vi "test Configuration Files Errors.vi"(8 "error in":errorcluster, 11 "TestCase in":refnum<class "Scripting.lvclass">) -> (0 "error out":errorcluster, 3 "TestCase out":refnum<class "Scripting.lvclass">)   [LabVIEW 2020, in "Scripting.lvclass"]
uses:
  Scripting.lvclass
  C:/dev/git/niveristand-custom-device-testing-tools/VeriStandScriptingTestCase/VeriStandScriptingTestCase.lvclass
  niveristand-custom-device-testing-tools/VeriStandScriptingTestCase/VeriStandScriptingTestCase.lvclass/VeriStandScriptingTestCase.ctl
  niveristand-custom-device-testing-tools/VeriStandScriptingTestCase/Read Target.vi
  Scripting/Constants.vi
  NationalInstruments.VeriStand.SystemDefinitionAPI
  <vilib>/addons/_JKI Toolkits/VI Tester/TestCase.llb/TestCase.lvclass
  Scripting/AIM MIL-STD-1553 Scripting.lvlib
  niveristand-custom-device-testing-tools/VeriStandTestUtilities/VeriStandTestUtilities.lvlib
  C:/Program Files (x86)/National Instruments/LabVIEW 2020/vi.lib/addons/_JKI Toolkits/VI Tester/TestCase.llb/TestCase.lvclass
  C:/dev/git/niveristand-aim-milStd1553-custom-device/Source/Custom Device Support/Tests/Unit/Scripting/Scripting.lvclass
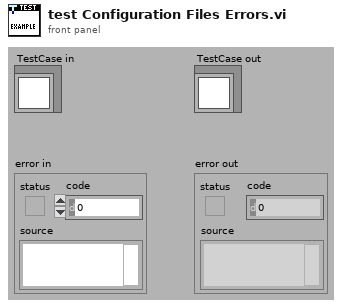
[diagram p1: front panel]
types:
  T1 = enum16{"open", "replace", "create", "open or create", "replace or create", "replace or create with confirmation"}
  T2 = typedef "Custom Device API.lvlib/Custom Device Item Ref.ctl" = u64
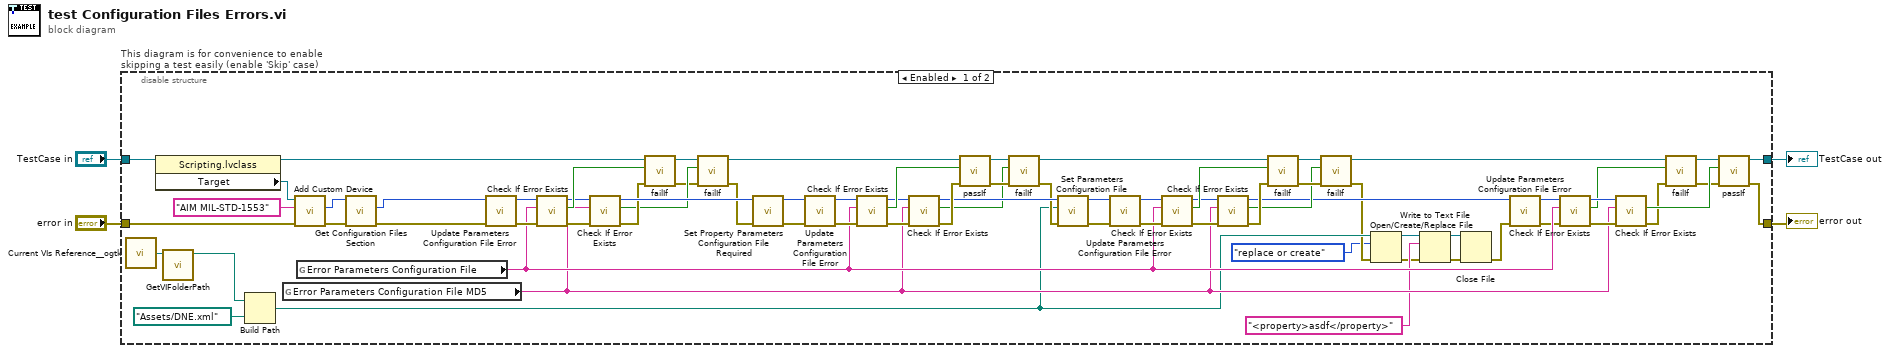
[diagram p0: block diagram]
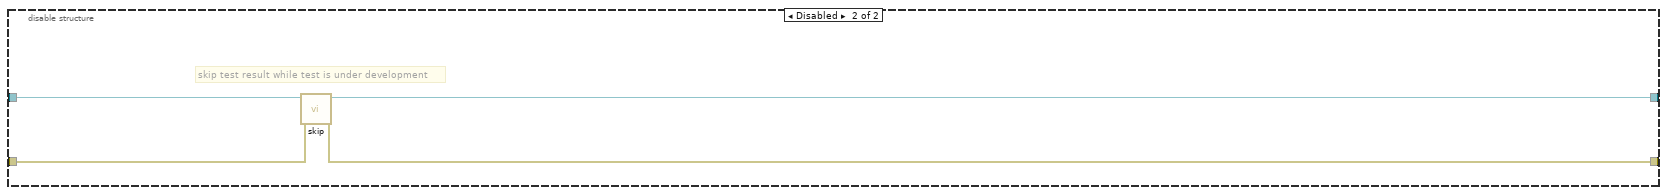
[diagram p2: hidden frame]
diagram:
  n1 = disable-structure "This diagram is for convenience to enable skipping a test easily (enable 'Skip' case)" shown="Enabled" {
    disable-tunnel: "TestCase in" -> [w75 w81]
    disable-tunnel: [w20 w79] -> w1
    disable-tunnel: [w19 w80] -> w3
    disable-tunnel: "error in" -> [w77 w78]
    frame Enabled {
      n2 = call <userlib>:"Current VIs Reference__ogtk.vi"() -> ("Current VI's reference"=w73:refnum<vi>)  [unwired: 5 in]
      n3 = property on="Property Node" class="Scripting.lvclass"(reference=w75) -> (reference out=w72:refnum<class "Scripting.lvclass">, "Target"=w74:refnum<k24>)  [unwired: 1 in, 1 out]
      n4 = call "GetVIFolderPath.vi"("VI Reference in"=w73) -> ("VI Folder Path out"=w59:path)  [unwired: 9 in, 1 out]
      n5 = Build Path(base path=w59, name or relative path=path "Assets/DNE.xml" ("hardware configuration file path")) -> (appended path=w11:path)
      n6 = global read "Constants.vi" "Error Parameters Configuration File MD5"() -> (w21:string)
      n7 = call "Add Custom Device.vi"("error in"=w77, "name"="AIM MIL-STD-1553", "target in"=w74) -> ("error out"=w67:errorcluster, "Ballard MIL-STD 1553 custom device"=w68:T2)  [unwired: 6 in, 1 out]
      n8 = global read "Constants.vi" "Error Parameters Configuration File"() -> (w22:string)
      n9 = call "Get Configuration Files Section.vi"("error in"=w67, "custom device in"=w68) -> ("error out"=w5:errorcluster, "configuration files section"=w6:T2)  [unwired: 6 in, 2 out]
      n10 = call "Update Parameters Configuration File Error.vi"("error in"=w5, "configuration files ref in"=w6) -> ("error out"=w71:errorcluster, "configuration files ref out"=w70:T2)  [unwired: 8 in]
      n11 = call "Check If Error Exists.vi"("error in"=w71, "error key"=w22, "section ref in"=w70) -> ("error out"=w53:errorcluster, "error exists?"=w69:bool, "section ref out"=w54:T2)  [unwired: 6 in]
      n12 = call "Check If Error Exists.vi"("error in"=w53, "error key"=w21, "section ref in"=w54) -> ("error out"=w51:errorcluster, "error exists?"=w50:bool, "section ref out"=w52:T2)  [unwired: 6 in]
      n13 = call-dynamic "failIf.vi"("error in (no error)"=w51, "fail"=w69, "TestCase in"=w72) -> ("error out"=w49:errorcluster, "TestCase out"=w48:refnum<class "Scripting.lvclass">)  [unwired: 7 in]
      n14 = call-dynamic "failIf.vi"("error in (no error)"=w49, "fail"=w50, "TestCase in"=w48) -> ("error out"=w47:errorcluster, "TestCase out"=w46:refnum<class "Scripting.lvclass">)  [unwired: 7 in]
      n15 = call "Set Property Parameters Configuration File Required.vi"("error in"=w47, "configuration files ref"=w52) -> ("error out"=w63:errorcluster, "configuration files ref out"=w64:T2)  [unwired: 8 in]
      n16 = call "Update Parameters Configuration File Error.vi"("error in"=w63, "configuration files ref in"=w64) -> ("error out"=w65:errorcluster, "configuration files ref out"=w66:T2)  [unwired: 8 in]
      n17 = call "Check If Error Exists.vi"("error in"=w65, "error key"=w22, "section ref in"=w66) -> ("error out"=w45:errorcluster, "error exists?"=w62:bool, "section ref out"=w44:T2)  [unwired: 6 in]
      n18 = call "Check If Error Exists.vi"("error in"=w45, "error key"=w21, "section ref in"=w44) -> ("error out"=w43:errorcluster, "error exists?"=w37:bool, "section ref out"=w42:T2)  [unwired: 6 in]
      n19 = call-dynamic "passIf.vi"("error in (no error)"=w43, "pass"=w62, "TestCase in"=w46) -> ("error out"=w40:errorcluster, "TestCase out"=w41:refnum<class "Scripting.lvclass">)  [unwired: 7 in]
      n20 = call-dynamic "failIf.vi"("error in (no error)"=w40, "fail"=w37, "TestCase in"=w41) -> ("error out"=w39:errorcluster, "TestCase out"=w38:refnum<class "Scripting.lvclass">)  [unwired: 7 in]
      n21 = call "Set Parameters Configuration File.vi"("error in"=w39, "parameters configuration file path"=w11, "Ballard MIL-STD 1553 custom device in"=w42) -> ("error out"=w56:errorcluster, "Ballard MIL-STD 1553 custom device out"=w57:T2)  [unwired: 7 in]
      n22 = call "Update Parameters Configuration File Error.vi"("error in"=w56, "configuration files ref in"=w57) -> ("error out"=w61:errorcluster, "configuration files ref out"=w60:T2)  [unwired: 8 in]
      n23 = call "Check If Error Exists.vi"("error in"=w61, "error key"=w22, "section ref in"=w60) -> ("error out"=w36:errorcluster, "error exists?"=w55:bool, "section ref out"=w35:T2)  [unwired: 6 in]
      n24 = call "Check If Error Exists.vi"("error in"=w36, "error key"=w21, "section ref in"=w35) -> ("error out"=w34:errorcluster, "error exists?"=w31:bool, "section ref out"=w15:T2)  [unwired: 6 in]
      n25 = call-dynamic "failIf.vi"("error in (no error)"=w34, "fail"=w55, "TestCase in"=w38) -> ("error out"=w32:errorcluster, "TestCase out"=w33:refnum<class "Scripting.lvclass">)  [unwired: 7 in]
      n26 = call-dynamic "failIf.vi"("error in (no error)"=w32, "fail"=w31, "TestCase in"=w33) -> ("error out"=w10:errorcluster, "TestCase out"=w23:refnum<class "Scripting.lvclass">)  [unwired: 7 in]
      n27 = Open/Create/Replace File(file path (use dialog)=w11, error in=w10, operation (0:open)=T1."replace or create") -> (refnum out=w9:refnum<file>, error out=w8:errorcluster)  [unwired: 3 in, 1 out]
      n28 = Write to Text File(file (use dialog)=w9, text="<property>asdf</property>", error in=w8) -> (refnum out=w17:refnum<file>, error out=w16:errorcluster)  [unwired: 1 in, 1 out]
      n29 = Close File(refnum=w17, error in=w16) -> (error out=w14:errorcluster)  [unwired: 1 out]
      n30 = call "Update Parameters Configuration File Error.vi"("error in"=w14, "configuration files ref in"=w15) -> ("error out"=w12:errorcluster, "configuration files ref out"=w13:T2)  [unwired: 8 in]
      n31 = call "Check If Error Exists.vi"("error in"=w12, "error key"=w22, "section ref in"=w13) -> ("error out"=w25:errorcluster, "error exists?"=w24:bool, "section ref out"=w26:T2)  [unwired: 6 in]
      n32 = call "Check If Error Exists.vi"("error in"=w25, "error key"=w21, "section ref in"=w26) -> ("error out"=w27:errorcluster, "error exists?"=w30:bool)  [unwired: 6 in, 1 out]
      n33 = call-dynamic "failIf.vi"("error in (no error)"=w27, "fail"=w24, "TestCase in"=w23) -> ("error out"=w29:errorcluster, "TestCase out"=w28:refnum<class "Scripting.lvclass">)  [unwired: 7 in]
      n34 = call-dynamic "passIf.vi"("error in (no error)"=w29, "pass"=w30, "TestCase in"=w28) -> ("error out"=w19:errorcluster, "TestCase out"=w20:refnum<class "Scripting.lvclass">)  [unwired: 7 in]
    }
    frame Disabled {
      # "skip test result while test is under development"
      n35 = call <vilib>:"skip.vi"("error in (no error)"=w78, "TestCase in"=w81) -> ("error out"=w80:errorcluster, "TestCase out"=w79:refnum<class "Scripting.lvclass">)  [unwired: 8 in]
    }
  }
  "error out" <- w3
  "TestCase out" <- w1
